vi "niScope Actual Record Length.vi"(0 "instrument handle":refnum<k15>, 11 "error in":errorcluster) -> (4 "instrument handle out":refnum<k15>, 8 "actual record length":i32, 15 "error out":errorcluster)   [LabVIEW 2013]
doc: "Returns the actual number of points the digitizer acquires for each channel. After configuring the digitizer for an acquisition, call this VI to determine the size of the waveforms that the digitizer acquires. The value is equal to or greater than the minimum number of points specified in any of the Configure Horizontal VIs."
uses:
  niScope_32.dll
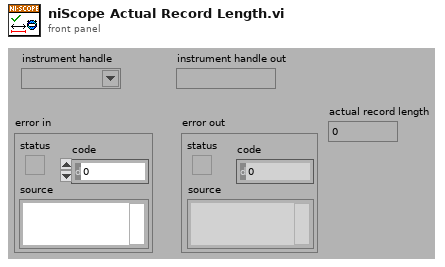
[diagram p1: front panel]
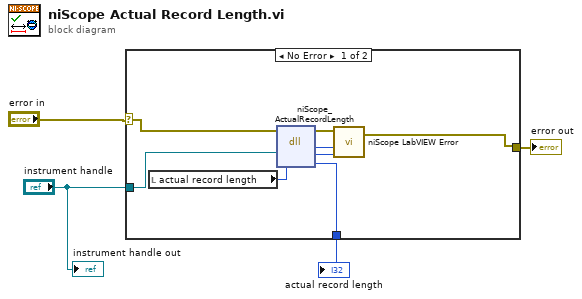
[diagram p0: block diagram]
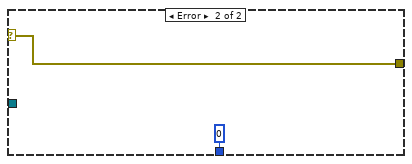
[diagram p2: hidden frame]
diagram:
  n1 = case shown="No Error" "error in" {
    selector: "error in" -> [w5 w12]
    tunnel: [w6 w12] -> w3
    tunnel: "instrument handle" -> [w11 _]
    tunnel: [w10 0 ("actual  record length")] -> w1
    frame No Error {
      n2 = local read "actual record length"() -> (w9:i32)
      n3 = dll-call lib="niScope_*.*" fn="niScope_ActualRecordLength"("instrument handle"=w11, "actualRecordLength"=w9) -> ("status"=w8:i32, "instrument handle"=w7:u32, "actualRecordLength"=w10:i32)  [unwired: 3 in, 2 out]
      n4 = call <instrlib>:"niScope LabVIEW Error.vi"("instrument handle"=w7, "niScope error code (0)"=w8, "error in (no error)"=w5) -> ("error out"=w6:errorcluster)  [unwired: 2 in]
    }
    frame Error {
    }
  }
  "error out" <- w3
  "actual record length" <- w1
  "instrument handle out" <- "instrument handle"
